vi "Delay Line.vi"() -> ()   [LabVIEW 2020]
uses:
  C:/Users/ssechi/Desktop/LabView Projects/Thorlabs.MotionControl.Controls.dll
  Thorlabs.MotionControl.Controls.dll
  C:/Users/ssechi/Desktop/LabView Projects/ThorLabs.MotionControl.KCube.DCServoCLI.dll
  ThorLabs.MotionControl.KCube.DCServoCLI.dll
  Global Position.vi
panel:
  in  "Define home":bool
  in  "Zero (mm)":dbl=-157036.0
  out "Actual position":dbl
  in  "-100 fs":bool
  in  "-1 ps":bool
  in  "-10ps":bool
  in  "-10 fs":bool
  in  "+10 ps":bool
  in  "+1 ps":bool
  in  "+100 fs":bool
  in  "+10 fs":bool
  in  "Move to (fs)":dbl
  in  "GO!!!":bool
  in  "STOP MOVEMENT":bool
  out "Current Position":dbl
  out "Step size 3":dbl
  out "Step size 2":dbl
  out "Step size 1":dbl
  in  "?":bool
  in  "Enable device movement":bool
  in  "START SCAN":bool
  in  "?":bool
  in  "SECOND INTERVAL":bool
  in  "THIRD INTERVAL":bool
  out "Position array":dbl[](array[numeric])
  in  "?":T1
  in  "?":T1
  in  "?":T2
  out "Device":refnum<k24>
  out "KCubeDCServoControl initialized":refnum<k24>
  out "DEVICE INITIALIZATION":bool
  # "fs"
  # "Translation STAGE"
  # "Move to new\nabsolute position..."
  # "SCANNING MEASUREMENTS"
  # "FIRST INTERVAL"
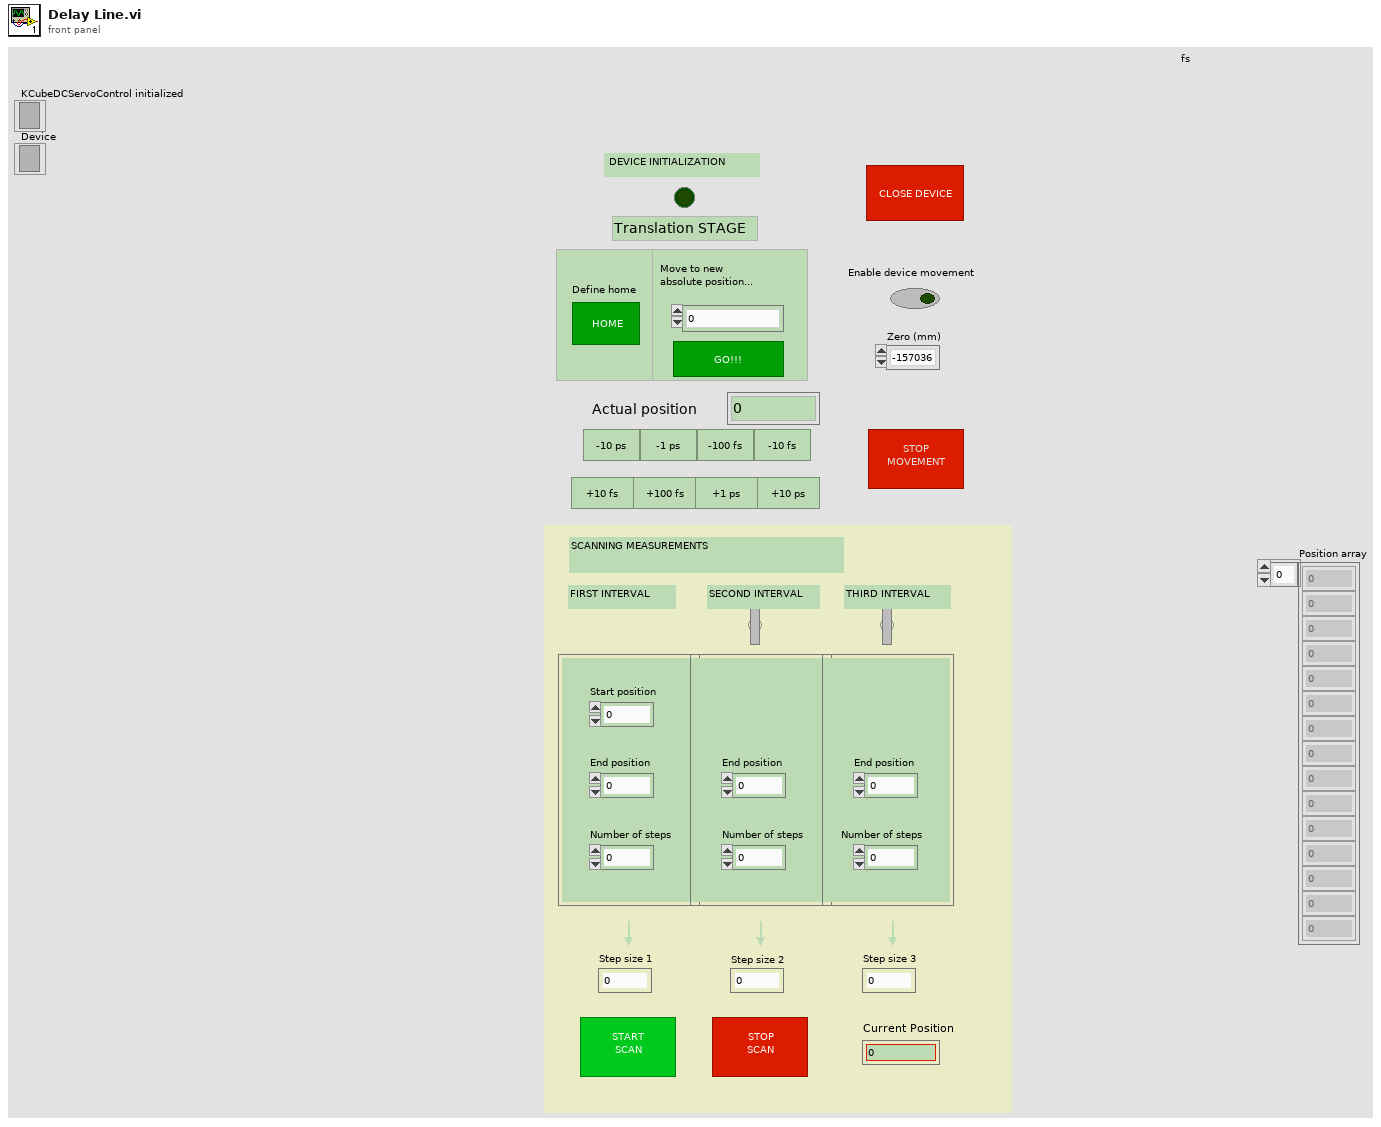
[diagram p1: front panel]
types:
  T1 = cluster{"Number of steps":dbl, "End position":dbl}
  T2 = cluster{"Number of steps ":dbl, "End position ":dbl, "Start position":dbl}
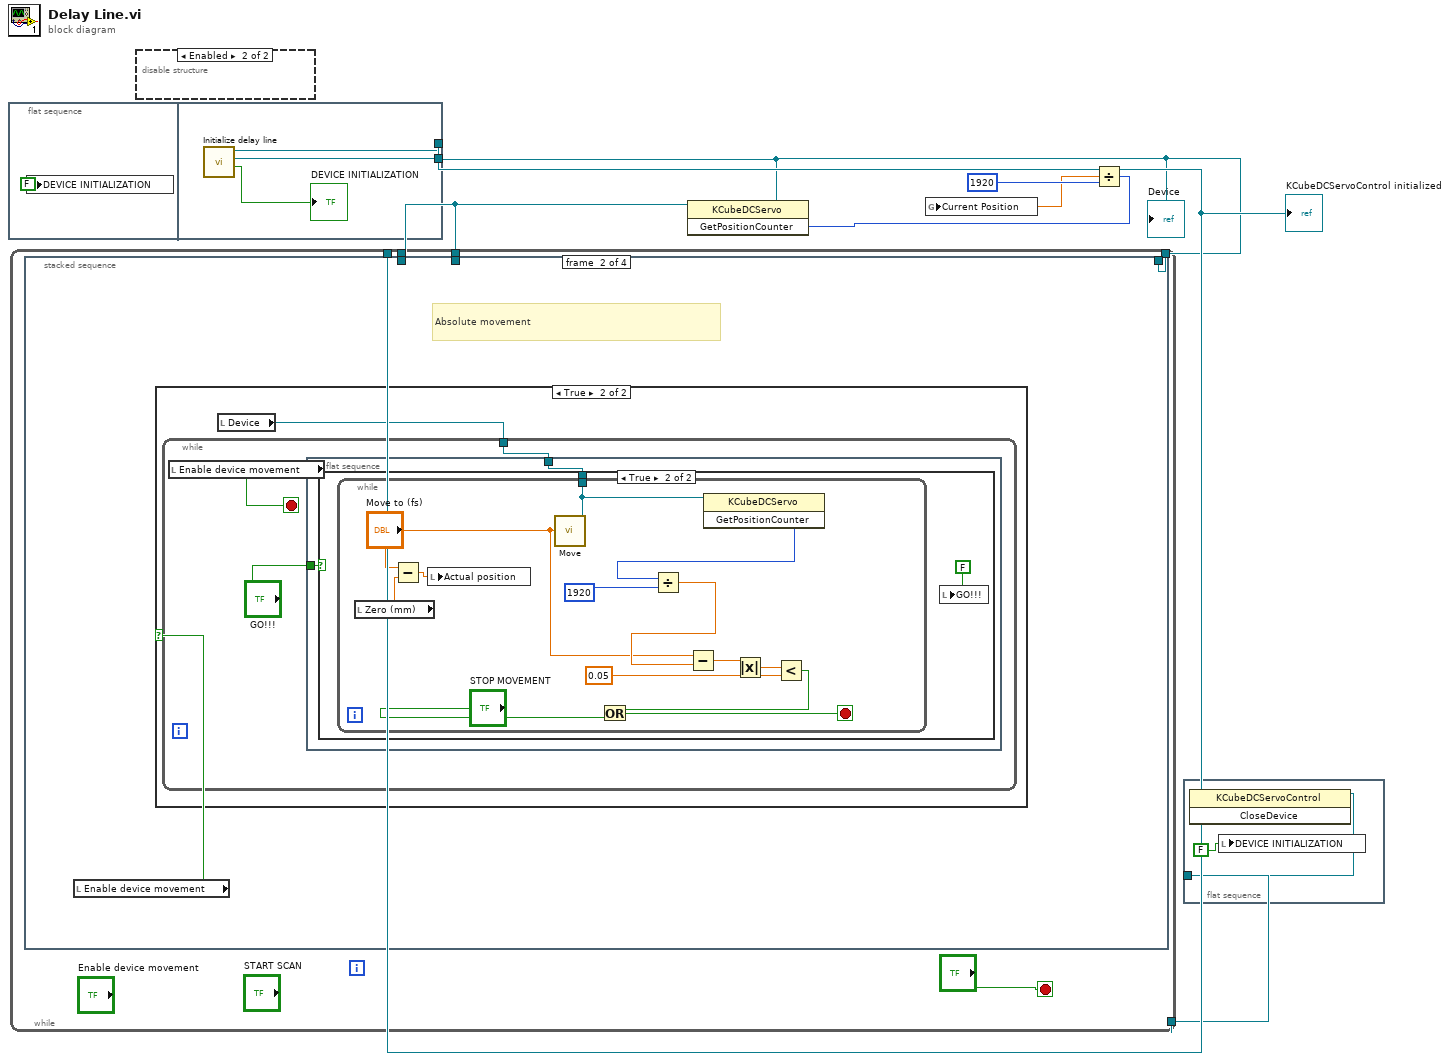
[diagram p0: block diagram]
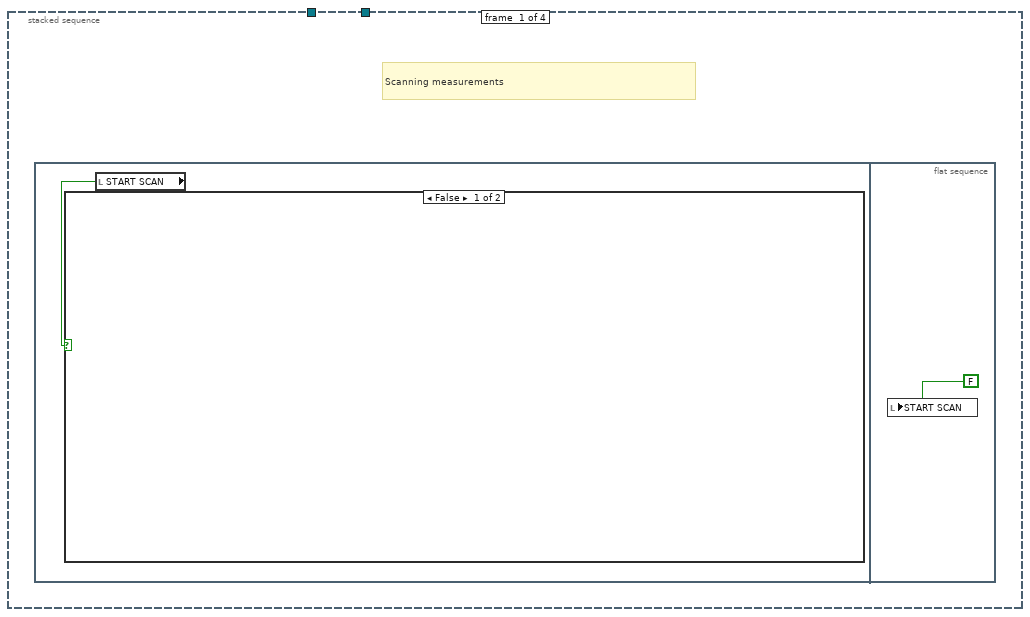
[diagram p3: hidden frame]
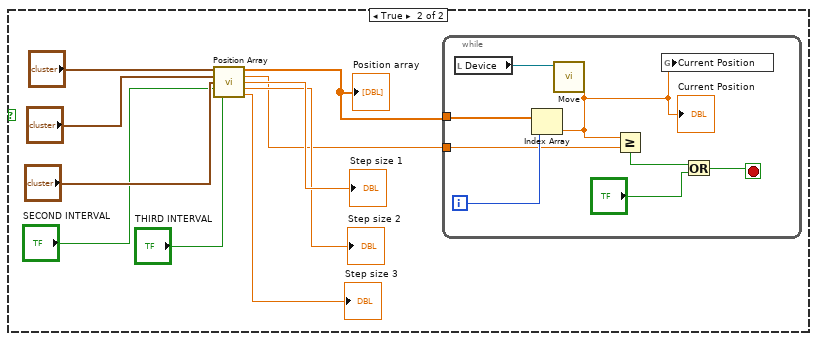
[diagram p4: hidden frame]
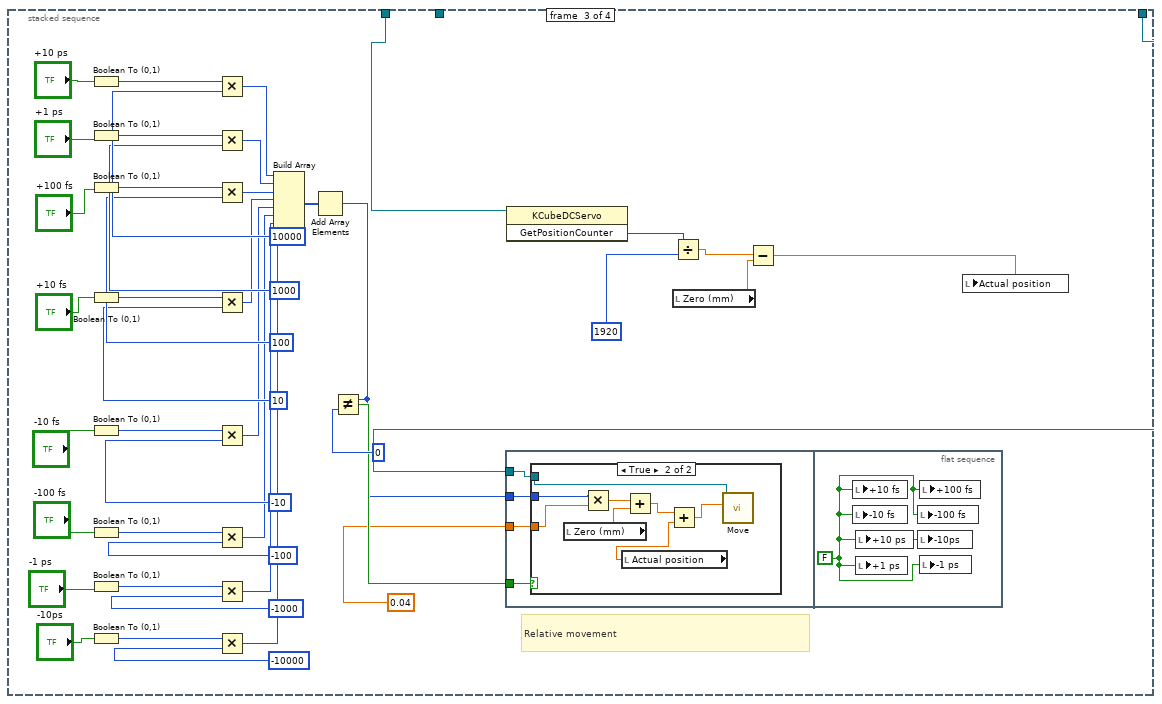
[diagram p7: hidden frame]
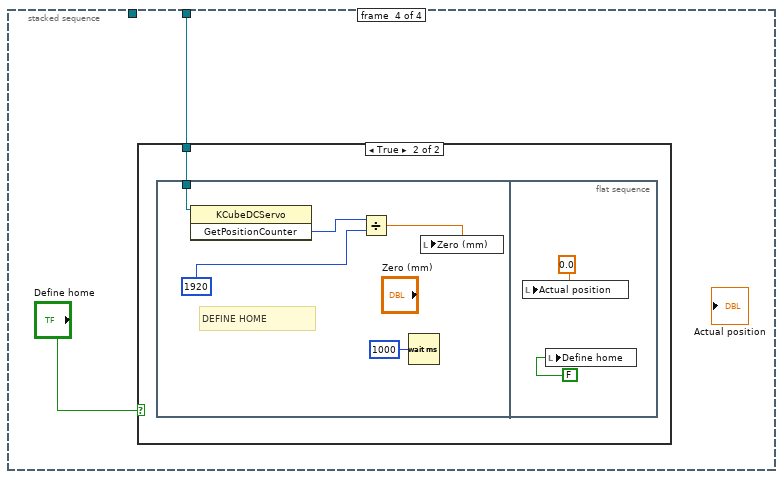
[diagram p9: hidden frame]
diagram:
  n1 = flat-sequence {
    tunnel: [w10] -> w6
    tunnel: [w9] -> w1
    frame #0 {
      n2 = local write "DEVICE INITIALIZATION"(FALSE ("Device initialized")) -> ()
    }
    frame #1 {
      n3 = call "Initialize delay line.vi"() -> ("Device initialized"=→"DEVICE INITIALIZATION":bool, "KCubeDCServoControl initialized"=w10:refnum<k24>, "Device"=w9:refnum<k24>)  [unwired: 9 in]
    }
  }
  n4 = while {
    tunnel: [w15] -> w3
    tunnel: w6 -> [w15]
    tunnel: w1 -> [w13]
    tunnel: w1 -> [w12]
    tunnel: w1 -> [w11]
    stop <- "?" stop-if-true
    n5 = stacked-sequence {
      tunnel: w13 -> [_ _ w61 _]
      tunnel: w12 -> [_ _ w64 _]
      tunnel: w11 -> [_ _ _ w115]
      frame #0 {
        # "Scanning measurements"
        n6 = flat-sequence {
          frame #0 {
            n7 = local read "START SCAN"() -> (w16:bool)
            n8 = case shown="False" w16 {
              frame False {
              }
              frame True {
                n9 = call "Position Array.vi"("First interval parameters"="?", "Second interval parameters"="?", "Third interval parameters"="?", "Second interval"="SECOND INTERVAL", "Third interval"="THIRD INTERVAL") -> ("Position array"=w18:dbl[], "End position"=w17:dbl, "Step size 1"=→"Step size 1":dbl, "Step size 2"=→"Step size 2":dbl, "Step size 3"=→"Step size 3":dbl)  [unwired: 6 in]
                "Position array" <- w18
                n10 = while {
                  tunnel: w18 -> [w33]
                  tunnel: w17 -> [w27]
                  i -> [w32]
                  stop <- w30 stop-if-true
                  n11 = local read "Device"() -> (w34:refnum<k24>)
                  n12 = Index Array(array=w33, index=w32) -> (element=w28:dbl)
                  "Current Position" <- w28
                  n13 = call "Move.vi"("position"=w28, "Device"=w34) -> ()  [unwired: 10 in]
                  n14 = Greater Or Equal?(x=w28, y=w27) -> (x >= y?=w29:bool)
                  n15 = global write "Global Position.vi" "Current Position"(w28) -> ()
                  n16 = Or(x=w29, y="?") -> (x .or. y?=w30:bool)
                }
              }
            }
          }
          frame #1 {
            n17 = local write "START SCAN"(FALSE ("START SCAN")) -> ()
          }
        }
      }
      frame #1 {
        # "Absolute movement"
        n18 = local read "Enable device movement"() -> (w36:bool)
        n19 = case shown="True" w36 {
          frame False {
          }
          frame True {
            n20 = local read "Device"() -> (w37:refnum<k24>)
            n21 = while {
              tunnel: w37 -> [w39]
              stop <- w40 stop-if-true
              n22 = local read "Enable device movement"() -> (w40:bool)
              n23 = flat-sequence {
                tunnel: "GO!!!" -> [w42]
                tunnel: w39 -> [w41]
                frame #0 {
                  n24 = case shown="True" w42 {
                    tunnel: w41 -> [_ w44]
                    frame False {
                    }
                    frame True {
                      n25 = while {
                        tunnel: w44 -> [w56]
                        stop <- w49 stop-if-true
                        n26 = local read "Zero (mm)"() -> (w46:dbl)
                        n27 = Subtract(x="Move to (fs)", y=w46) -> (x-y=w45:dbl)
                        n28 = local write "Actual position"(w45) -> ()
                        n29 = call "Move.vi"("position"="Move to (fs)", "Device"=w56) -> ()  [unwired: 10 in]
                        n30 = invoke class="KCubeDCServo" method="GetPositionCounter"(reference=w56) -> ("GetPositionCounter"=w55:i32)  [unwired: 2 in, 2 out]
                        n31 = Divide(x=w55, y=1920) -> (x/y=w48:dbl)
                        n32 = Subtract(x="Move to (fs)", y=w48) -> (x-y=w53:dbl)
                        n33 = Absolute Value(x=w53) -> (abs(x)=w52:dbl)
                        n34 = Less?(x=w52, y=0.05) -> (x < y?=w50:bool)
                        n35 = Or(x=w50, y="STOP MOVEMENT") -> (x .or. y?=w49:bool)
                      }
                      n36 = local write "GO!!!"(FALSE ("Move device")) -> ()
                    }
                  }
                }
              }
            }
          }
        }
      }
      frame #2 {
        # "Relative movement"
        n37 = Boolean To (0,1)(Boolean="+10 ps") -> (0, 1=w101:i16)
        n38 = Boolean To (0,1)(Boolean="+1 ps") -> (0, 1=w99:i16)
        n39 = Boolean To (0,1)(Boolean="+100 fs") -> (0, 1=w96:i16)
        n40 = Boolean To (0,1)(Boolean="+10 fs") -> (0, 1=w95:i16)
        n41 = Boolean To (0,1)(Boolean="-10 fs") -> (0, 1=w92:i16)
        n42 = Boolean To (0,1)(Boolean="-100 fs") -> (0, 1=w91:i16)
        n43 = Boolean To (0,1)(Boolean="-1 ps") -> (0, 1=w88:i16)
        n44 = Boolean To (0,1)(Boolean="-10ps") -> (0, 1=w87:i16)
        n45 = Multiply(x=w101, y=10000) -> (x*y=w82:i32)
        n46 = Multiply(x=w99, y=1000) -> (x*y=w83:i32)
        n47 = Multiply(x=w96, y=100) -> (x*y=w84:i32)
        n48 = Multiply(x=w95, y=10) -> (x*y=w85:i32)
        n49 = Multiply(x=w92, y=-10) -> (x*y=w81:i32)
        n50 = Multiply(x=w91, y=-100) -> (x*y=w80:i32)
        n51 = Multiply(x=w88, y=-1000) -> (x*y=w79:i32)
        n52 = Multiply(x=w87, y=-10000) -> (x*y=w78:i32)
        n53 = Build Array(w82, w83, w84, w85, w81, w80, w79, w78) -> (w76:i32[])
        n54 = Add Array Elements(numeric array=w76) -> (sum=w68:i32)
        n55 = Not Equal?(x=w68, y=0) -> (x != y?=w69:bool)
        n56 = flat-sequence {
          tunnel: w69 -> [w105]
          tunnel: w68 -> [w104]
          tunnel: 0.04 -> [w103]
          tunnel: w61 -> [w102]
          frame #0 {
            n57 = case shown="True" w105 {
              tunnel: w104 -> [_ w112]
              tunnel: w103 -> [_ w111]
              tunnel: w102 -> [_ w113]
              frame False {
              }
              frame True {
                n58 = local read "Zero (mm)"() -> (w109:dbl)
                n59 = Multiply(x=w112, y=w111) -> (x*y=w110:dbl)
                n60 = local read "Actual position"() -> (w106:dbl)
                n61 = Add(x=w110, y=w109) -> (x+y=w108:dbl)
                n62 = Add(x=w108, y=w106) -> (x+y=w107:dbl)
                n63 = call "Move.vi"("position"=w107, "Device"=w113) -> ()  [unwired: 10 in]
              }
            }
          }
          frame #1 {
            w114 = FALSE ("+10 fs")
            n64 = local write "+10 fs"(w114) -> ()
            n65 = local write "-10 fs"(w114) -> ()
            n66 = local write "+10 ps"(w114) -> ()
            n67 = local write "+1 ps"(w114) -> ()
            n68 = local write "-100 fs"(w114) -> ()
            n69 = local write "-10ps"(w114) -> ()
            n70 = local write "+100 fs"(w114) -> ()
            n71 = local write "-1 ps"(w114) -> ()
          }
        }
        n72 = invoke class="KCubeDCServo" method="GetPositionCounter"(reference=w64) -> ("GetPositionCounter"=w66:i32)  [unwired: 2 in, 2 out]
        n73 = Divide(x=w66, y=1920) -> (x/y=w63:dbl)
        n74 = local read "Zero (mm)"() -> (w65:dbl)
        n75 = Subtract(x=w63, y=w65) -> (x-y=w60:dbl)
        n76 = local write "Actual position"(w60) -> ()
      }
      frame #3 {
        n77 = case shown="True" "Define home" {
          tunnel: w115 -> [_ w117]
          frame False {
          }
          frame True {
            n78 = flat-sequence {
              tunnel: w117 -> [w119]
              frame #0 {
                # "DEFINE HOME"
                n79 = invoke class="KCubeDCServo" method="GetPositionCounter"(reference=w119) -> ("GetPositionCounter"=w118:i32)  [unwired: 2 in, 2 out]
                n80 = Divide(x=w118, y=1920) -> (x/y=w121:dbl)
                n81 = Wait (ms)(milliseconds to wait=u32 1000) -> ()  [unwired: 1 out]
                n82 = local write "Zero (mm)"(w121) -> ()
              }
              frame #1 {
                n83 = local write "Actual position"(0.0 ("Actual position")) -> ()
                n84 = local write "Define home"(FALSE ("Define HOME")) -> ()
              }
            }
          }
        }
      }
    }
  }
  n85 = disable-structure shown="Enabled" {
    frame Disabled {
      # "Device initialization"
    }
    frame Enabled {
    }
  }
  n86 = invoke class="KCubeDCServo" method="GetPositionCounter"(reference=w1) -> ("GetPositionCounter"=w2:i32)  [unwired: 2 in, 2 out]
  n87 = Divide(x=w2, y=1920) -> (x/y=w4:dbl)
  n88 = global write "Global Position.vi" "Current Position"(w4) -> ()
  n89 = flat-sequence {
    tunnel: w3 -> [w126]
    frame #0 {
      n90 = invoke class="KCubeDCServoControl" method="CloseDevice"(reference=w126) -> ()  [unwired: 2 in, 3 out]
      n91 = local write "DEVICE INITIALIZATION"(FALSE) -> ()
    }
  }
  "KCubeDCServoControl initialized" <- w6
  "Device" <- w1
